vi "Configure Serial Bus (CAN - Basic).vi"(0 "VISA resource name":refnum<visa-resource-name>, 5 "Serial Bus Name (1: Serial Bus 1)":i32(ring)=1 items=["Serial Bus 1"=1, "Serial Bus 2"=2], 7 "Baudrate (125000 bps)":i32=125000, 9 "Source (0: Channel 1)":i32(ring) items=["Channel 1"=0, "Channel 2"=1, "Channel 3"=2, "Channel 4"=3, "D0"=13, "D1"=14, "D2"=15, "D3"=16, "D4"=17, "D5"=18, "D6"=19, "D7"=20, "D8"=21, "D9"=22, "D10"=23, "D11"=24, "D12"=25, "D13"=26, "D14"=27, "D15"=28, "External"=29], 11 "error in (no error)":errorcluster, 12 "Sample Point (60 percents)":dbl=60.0) -> (4 "VISA resource name out":refnum<visa-resource-name>, 15 "error out":errorcluster)   [LabVIEW 2023, in "Keysight-DSQx3014T.lvlib"]
doc: "Configures the basic settings of CAN bus."
uses:
  Keysight-DSQx3014T.lvlib
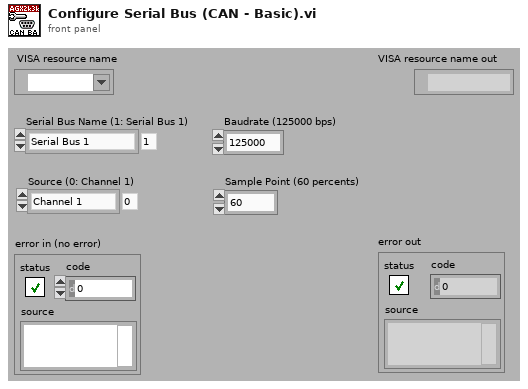
[diagram p1: front panel]
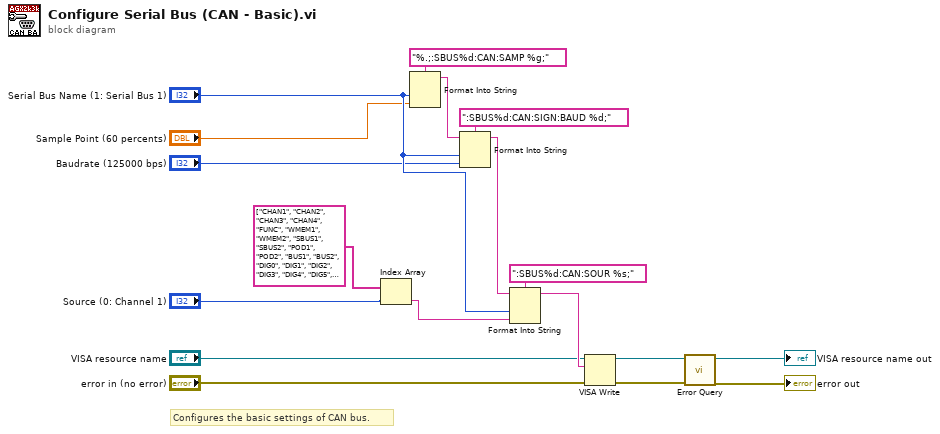
[diagram p0: block diagram]
diagram:
  # "Configures the basic settings of CAN bus."
  n1 = Index Array(array=string[] ["CHAN1", "CHAN2", "CHAN3", "CHAN4", "FUNC", "WMEM1", "WMEM2", "SBUS1", "SBUS2", "POD1", "POD2", "BUS1", "BUS2", "DIG0", "DIG1", "DIG2", "DIG3", "DIG4", "DIG5", "DIG6", "DIG7", "DIG8", "DIG9", "DIG10", "DIG11", "DIG12", "DIG13", "DIG14", "DIG15", "EXT", "LINE", "WGEN"], index="Source (0: Channel 1)") -> (element=w1:string)
  n2 = Format Into String(format string="%.;:SBUS%d:CAN:SAMP %g;", "Serial Bus Name (1: Serial Bus 1)", "Sample Point (60 percents)") -> (resulting string=w15:string)  [unwired: 2 in, 1 out]
  n3 = Format Into String(format string=":SBUS%d:CAN:SIGN:BAUD %d;", initial string=w15, "Serial Bus Name (1: Serial Bus 1)", "Baudrate (125000 bps)") -> (resulting string=w12:string)  [unwired: 1 in, 1 out]
  n4 = Format Into String(format string=":SBUS%d:CAN:SOUR %s;", initial string=w12, "Serial Bus Name (1: Serial Bus 1)", w1) -> (resulting string=w10:string)  [unwired: 1 in, 1 out]
  n5 = VISA Write(VISA resource name="VISA resource name", write buffer=w10, error in (no error)="error in (no error)") -> (VISA resource name out=w7:refnum<visa-resource-name>, error out=w6:errorcluster)  [unwired: 1 out]
  n6 = call "Error Query.vi"("error in (no error)"=w6, "VISA resource name"=w7) -> ("error out"=→"error out":errorcluster, "VISA resource name out"=→"VISA resource name out":refnum<visa-resource-name>)  [unwired: 8 out]
